vi "VsEP Write Cal Data.vi"(0 "Atten (dB)":dbl[](array[numeric]), 1 "Params":T4, 2 "Data Folder":path, 5 "accelerometer (mV)":dbl[](array[numeric]), 7 "Sensitivity":dbl, 11 "error in (no error)":errorcluster, 12 "Linear":dbl[][](array[numeric]), 13 "Nonlinear":dbl[][](array[numeric])) -> (15 "error out":errorcluster)   [LabVIEW 2020]
uses:
  Typedefs/VsEPCal- Stimulus.ctl
  Typedefs/VsEP-Hidden Params.ctl
  epl-vi-lib/Signal Synthesis VIs/Controls/Gate XCtl/Gate Control.xctl
panel:
  in  "VsEP Calibration Data File":T1
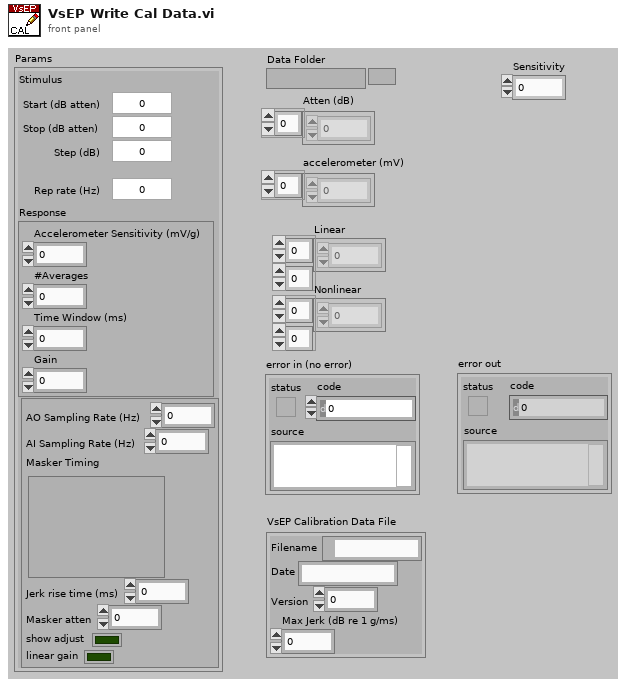
[diagram p1: front panel]
types:
  T1 = cluster{"Filename":path, "Date":string, "Version":i32, "Max Jerk (dB re 1 g/ms)":dbl}
  T2 = typedef "VsEPCal- Stimulus.ctl" = cluster{"Rep rate (Hz)":dbl, "Start (dB atten)":dbl, "Stop (dB atten)":dbl, "Step (dB)":dbl}
  T3 = typedef "VsEP-Hidden Params.ctl" = cluster{"AO Sampling Rate (Hz)":dbl, "AI Sampling Rate (Hz)":dbl, "Masker Timing":cluster{"Active":bool, "Delay (ms)":dbl, "Width (ms)":dbl, "Ramp (ms)":dbl}, "Jerk rise time (ms)":dbl, "Masker atten":dbl, "show adjust":bool, "linear gain":bool}
  T4 = cluster{"Stimulus":T2, "Response":cluster{"Accelerometer Sensitivity (mV/g)":dbl, "#Averages":i32, "Time Window (ms)":dbl, "Gain":dbl}, "Hidden":T3}
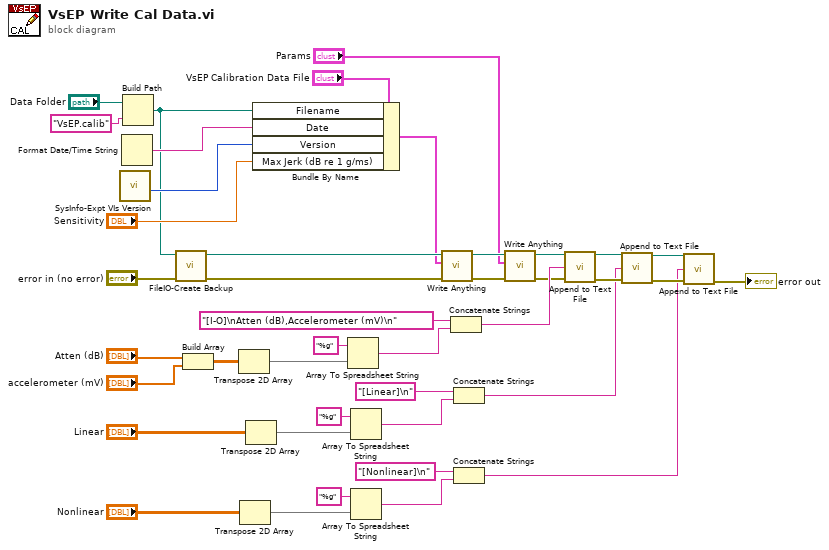
[diagram p0: block diagram]
diagram:
  n1 = call "SysInfo-Expt VIs Version.vi"() -> ("Expt VIs Version out"=w31:i32)  [unwired: 11 in]
  n2 = Format Date/Time String() -> (date/time string=w32:string)  [unwired: 3 in]
  n3 = Build Path(base path="Data Folder", name or relative path="VsEP.calib" ("tag")) -> (appended path=w29:path)
  n4 = call "FileIO-Create Backup.vi"("error in (no error)"="error in (no error)", "Path"=w29) -> ("error out"=w25:errorcluster, "Path (thru)"=w27:path)  [unwired: 6 in, 2 out]
  n5 = Build Array("Atten (dB)", "accelerometer (mV)") -> (w37:dbl[][])
  n6 = Transpose 2D Array(2D array=w37) -> (transposed array=w34:dbl[][])
  n7 = Transpose 2D Array(2D array="Nonlinear") -> (transposed array=w1:dbl[][])
  n8 = Transpose 2D Array(2D array="Linear") -> (transposed array=w2:dbl[][])
  n9 = Bundle By Name(cluster="VsEP Calibration Data File", "Filename"=w29, "Date"=w32, "Version"=w31, "Max Jerk (dB re 1 g/ms)"="Sensitivity") -> (w26:T1)
  n10 = Array To Spreadsheet String(array=w34, 3:"%g" ("format string")) -> (spreadsheet string=w36:string)  [unwired: 1 in]
  n11 = Array To Spreadsheet String(array=w2, 3:"%g" ("format string")) -> (spreadsheet string=w12:string)  [unwired: 1 in]
  n12 = Array To Spreadsheet String(array=w1, 3:"%g" ("format string")) -> (spreadsheet string=w7:string)  [unwired: 1 in]
  n13 = call "Write Anything.vi"("Error In"=w25, "Anything"=w26, "Path (dialog)"=w27) -> ("Error Out"=w21:errorcluster, "Path out"=w22:path)  [unwired: 7 in]
  n14 = Concatenate Strings("[I-O]\nAtten (dB),Accelerometer (mV)\n" ("format string"), w36) -> (w23:string)
  n15 = Concatenate Strings("[Linear]\n" ("format string"), w12) -> (w8:string)
  n16 = Concatenate Strings("[Nonlinear]\n" ("format string"), w7) -> (w3:string)
  n17 = call "Write Anything.vi"("Error In"=w21, "Anything"="Params", "Path (dialog)"=w22) -> ("Error Out"=w19:errorcluster, "Path out"=w18:path)  [unwired: 7 in]
  n18 = call "Append to Text File.vi"("file path"=w18, "text"=w23, "error in (no error)"=w19) -> ("file path out"=w17:path, "error out"=w16:errorcluster)  [unwired: 11 in]
  n19 = call "Append to Text File.vi"("file path"=w17, "text"=w8, "error in (no error)"=w16) -> ("file path out"=w15:path, "error out"=w14:errorcluster)  [unwired: 11 in]
  n20 = call "Append to Text File.vi"("file path"=w15, "text"=w3, "error in (no error)"=w14) -> ("error out"=→"error out":errorcluster)  [unwired: 11 in, 1 out]
